vi "Generate Server RPC Messages.vi"(5 "Enum Metadata":T1[](array[typedef]), 7 "Messages Metadata":T2[](array[typedef]), 8 "error in (no error)":errorcluster, 11 "Library in":refnum<vi>) -> (0 "error out":errorcluster, 3 "Library out":refnum<vi>)   [LabVIEW 2019, in "gRPC Template Creation Utility.lvlib"]
uses:
  gRPC Template Creation Utility.lvlib
  TypeDefs/Message Metadata (Scripting).ctl
  TypeDefs/Message Element Metadata (Scripting).ctl
  TypeDefs/Message Element Type.ctl
  TypeDefs/Enum Metadata (Scripting).ctl
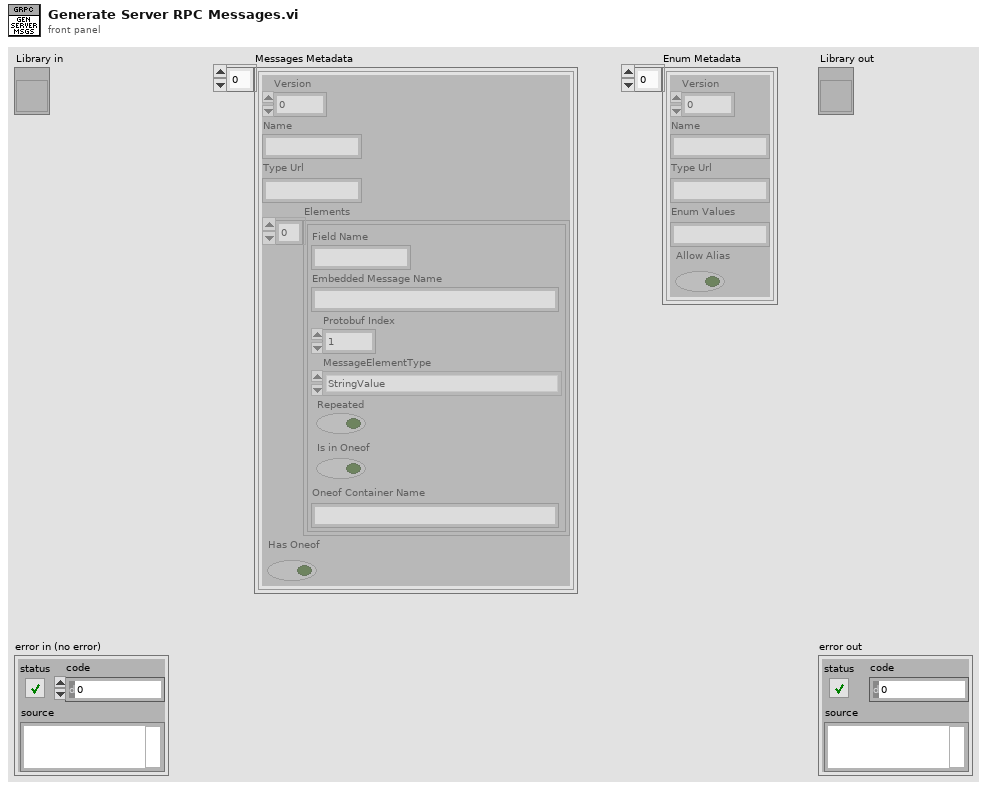
[diagram p1: front panel]
types:
  T1 = typedef "gRPC Template Creation Utility.lvlib/Enum Metadata (Scripting).ctl" = cluster{"Version":i32, "Name":string, "Type Url":string, "Enum Values":string, "Allow Alias":bool}
  T2 = typedef "gRPC Template Creation Utility.lvlib/Message Metadata (Scripting).ctl" = cluster{"Version":i32, "Name":string, "Type Url":string, "Elements":T3[], "Has Oneof":bool}
  T3 = typedef "gRPC Template Creation Utility.lvlib/Message Element Metadata (Scripting).ctl" = cluster{"Field Name":string, "Embedded Message Name":string, "Protobuf Index":i32, "MessageElementType":T4, "Repeated":bool, "Is in Oneof":bool, "Oneof Container Name":string}
  T4 = typedef "gRPC Template Creation Utility.lvlib/Message Element Type.ctl" = enum32{"Int32Value", "FloatValue", "DoubleValue", "BoolValue", "StringValue", "MessageValue", "Int64Value", "UInt32Value", "UInt64Value", "EnumValue", "Bytes", "Fixed64", "Fixed32", "SFixed64", "SFixed32", "SInt64", "SInt32"}
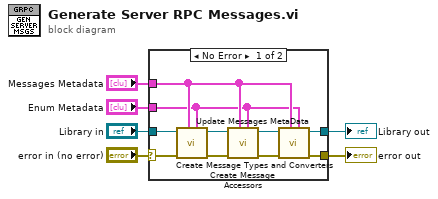
[diagram p0: block diagram]
diagram:
  n1 = case shown="No Error" "error in (no error)" {
    selector: "error in (no error)" -> [w14 w18]
    tunnel: [w13 w18] -> w6
    tunnel: [w9 w17] -> w5
    tunnel: "Messages Metadata" -> [w8 _]
    tunnel: "Library in" -> [w12 w17]
    tunnel: "Enum Metadata" -> [w7 _]
    frame No Error {
      n2 = call "Create Message Types and Converters.vi"("Enum parameters"=w7, "Message parameters"=w8, "error in (no error)"=w14, "Library in"=w12) -> ("error out"=w15:errorcluster, "Library out"=w16:refnum<vi>)  [unwired: 6 in]
      n3 = call "Create Message Accessors.vi"("enum parameters"=w7, "message parameters"=w8, "error in (no error)"=w15, "library in"=w16) -> ("error out"=w11:errorcluster, "library out"=w10:refnum<vi>)  [unwired: 6 in]
      n4 = call "Update Messages MetaData.vi"("enum metadata"=w7, "messages metadata"=w8, "error in (no error)"=w11, "library in"=w10) -> ("error out"=w13:errorcluster, "library out"=w9:refnum<vi>)  [unwired: 6 in]
    }
    frame Error {
    }
  }
  "error out" <- w6
  "Library out" <- w5
